vi "getScanName.vi"(8 "error in (no error)":errorcluster, 11 "Model in":refnum<class "Model.lvclass">) -> (0 "error out":errorcluster, 2 "Scan Name":string, 3 "Model out":refnum<class "Model.lvclass">)   [LabVIEW 2015, in "Model.lvclass"]
uses:
  Model.lvclass
  Model.lvclass/Model.ctl
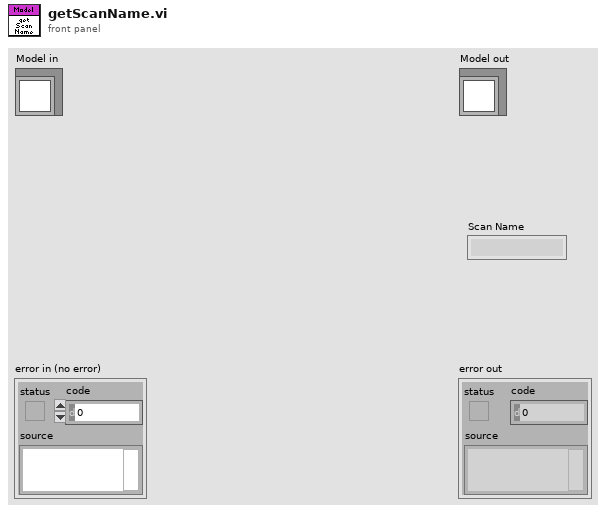
[diagram p1: front panel]
types:
  T1 = typedef "FAMTTypedefs.lvlib/Waveform.ctl" = enum16{"Sine Wave", "Triangle Wave", "Square Wave", "Sawtooth Wave", "Chirp Wave", "Gaussian Wave"}
  T2 = typedef "ILCCommon.lvlib/ILCConfiguration.lvlib/Scan Rates.ctl" = enum16{"50", "60", "100", "120", "200", "240", "300", "400", "480", "600", "1200", "2400", "4800"}
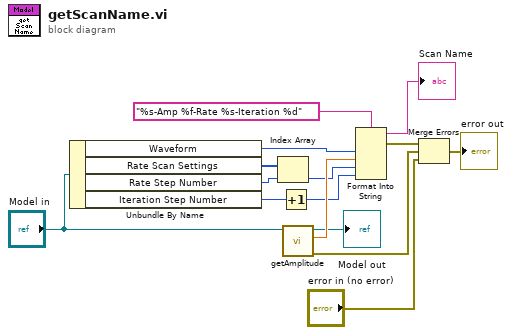
[diagram p0: block diagram]
diagram:
  n1 = Unbundle By Name("Model in") -> ("Waveform"=w14:T1, "Rate Scan Settings"=w12:T2[], "Rate Step Number"=w11:u16, "Iteration Step Number"=w2:u16)
  n2 = Index Array(array=w12, index=w11) -> (element=w10:T2)
  n3 = Increment(x=w2) -> (x+1=w1:u16)
  n4 = call "getAmplitude.vi"("Model in"="Model in") -> ("error out"=w5:errorcluster, "Result"=w13:dbl, "Model out"=→"Model out":refnum<class "Model.lvclass">)  [unwired: 8 in]
  n5 = Format Into String(format string="%s-Amp %f-Rate %s-Iteration %d", w14, w13, w10, w1) -> (resulting string=→"Scan Name":string, error out=w4:errorcluster)  [unwired: 2 in]
  n6 = Merge Errors(w4, w5, "error in (no error)") -> (→"error out":errorcluster)
